vi "Get_Ini_File_Paths.vi"(2 "Error in":errorcluster) -> (0 "Error out":errorcluster)   [LabVIEW 2013]
uses:
  Globals/Ini_Files.vi
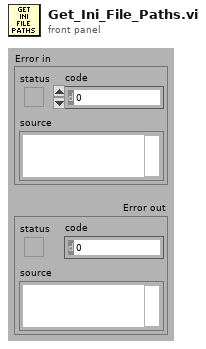
[diagram p1: front panel]
types:
  T1 = cluster{"Path Run Status file":path, "Path Default Settings file":path, "Path User Settings file":path}
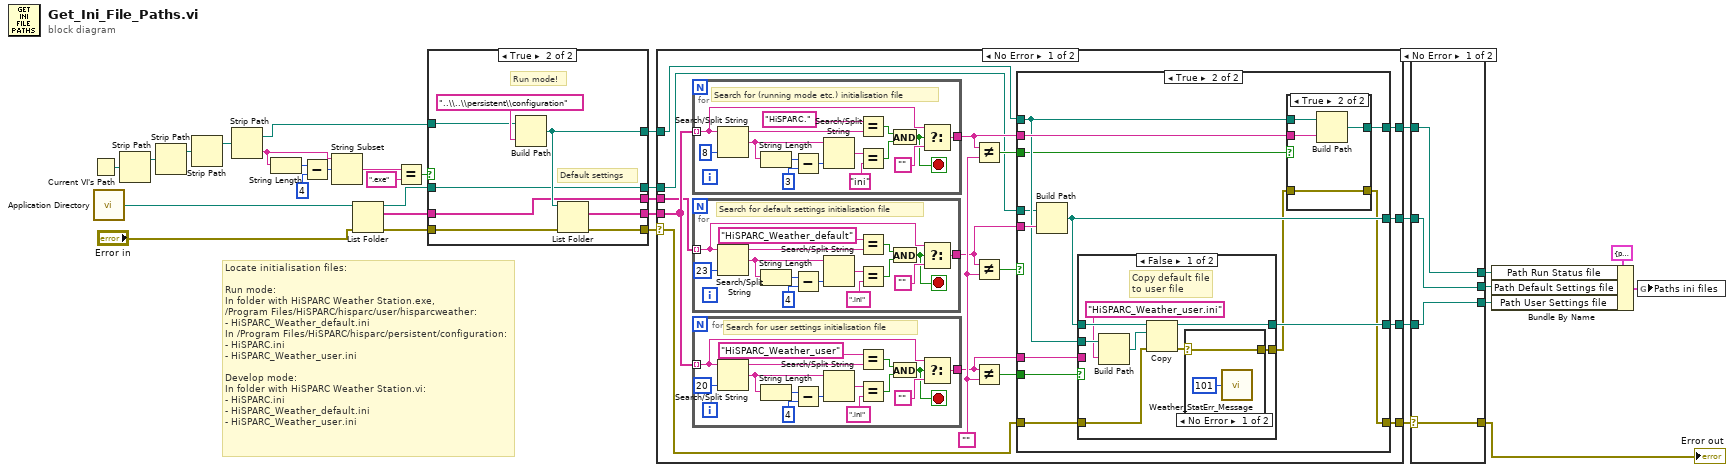
[diagram p0: block diagram]
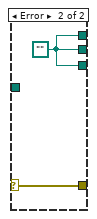
[diagram p3: hidden frame]
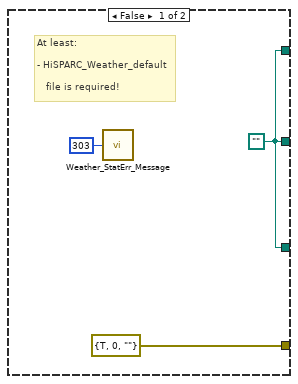
[diagram p4: hidden frame]
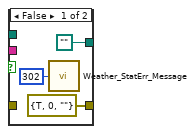
[diagram p5: hidden frame]
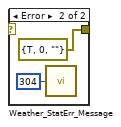
[diagram p6: hidden frame]
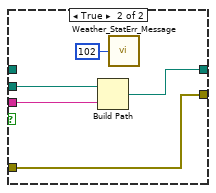
[diagram p7: hidden frame]
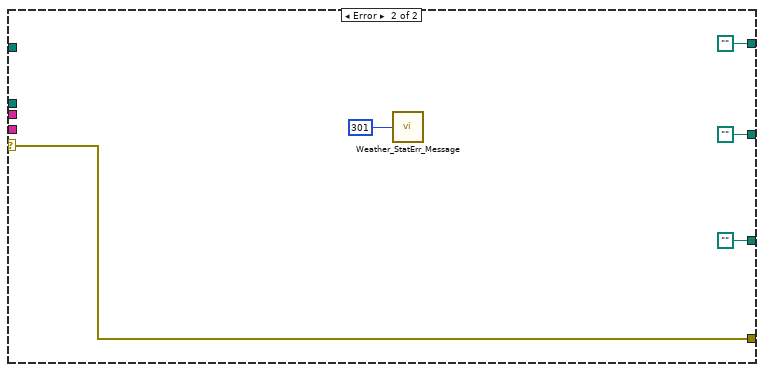
[diagram p8: hidden frame]
diagram:
  # "Locate initialisation files:\n\nRun mode:\nIn folder with HiSPARC Weather Station.exe,\n/Program Files/HiSPARC/hisparc/user/hisparcweather:\n- HiSPARC_Weather_default.ini\nIn /Program Files/HiSPARC/hisparc/persistent/configuration:\n- HiSPARC.ini\n- HiSPARC_Weather_user.ini\n\nDevelop mode:\nIn folder with HiSPARC Weather Station.vi:\n- HiSPARC.ini\n- HiSPARC_Weather_default.ini\n- HiSPARC_Weather_user.ini"
  n1 = Current VI's Path() -> (path=w7:path)
  n2 = call <vilib>:"Application Directory.vi"() -> ("Application Directory"=w8:path)
  n3 = Strip Path(path=w7) -> (stripped path=w6:path)  [unwired: 1 out]
  n4 = Strip Path(path=w6) -> (stripped path=w5:path)  [unwired: 1 out]
  n5 = Strip Path(path=w5) -> (stripped path=w3:path)  [unwired: 1 out]
  n6 = Strip Path(path=w3) -> (stripped path=w2:path, name=w4:string)
  n7 = String Length(string=w4) -> (length=w23:i32)
  n8 = Subtract(x=w23, y=4) -> (x-y=w21:i32)
  n9 = String Subset(string=w4, offset (0)=w21) -> (substring=w20:string)  [unwired: 1 in]
  n10 = List Folder(path=w8, error in="Error in") -> (path out=w15:path, filenames=w17:string[], error out=w14:errorcluster)  [unwired: 2 in, 1 out]
  n11 = Equal?(x=w20, y=".exe") -> (x = y?=w18:bool)
  n12 = case shown="True" w18 {
    tunnel: w17 -> [w33 w37]
    tunnel: w2 -> [_ w42]
    tunnel: w15 -> [w34 w39]
    tunnel: [w33 w36] -> w12
    tunnel: [w34 w39] -> w9
    tunnel: w14 -> [w35 w41]
    tunnel: [w35 w38] -> w13
    tunnel: [w34 w40] -> w10
    tunnel: [w33 w37] -> w11
    frame False {
      # "Develop mode!"
    }
    frame True {
      # "Default settings"
      # "Run mode!"
      n13 = Build Path(base path=w42, name or relative path="..\\..\\persistent\\configuration") -> (appended path=w40:path)
      n14 = List Folder(path=w40, error in=w41) -> (filenames=w36:string[], error out=w38:errorcluster)  [unwired: 2 in, 2 out]
    }
  }
  n15 = case shown="No Error" w13 {
    selector: w13 -> [w48 w146]
    tunnel: [w54 path "" ("Not A Path Constant")] -> w30
    tunnel: [w53 path ""] -> w32
    tunnel: [w52 path ""] -> w31
    tunnel: w12 -> [w47 _]
    tunnel: [w49 w146] -> w25
    tunnel: w11 -> [w46 _]
    tunnel: w10 -> [w45 _]
    tunnel: w9 -> [w44 _]
    frame No Error {
      w59 = ""
      n16 = for {
        tunnel: w47 -> [w92] mode=indexing
        tunnel: [w104] -> w56
        stop <- w93 stop-if-true
        # "Search for (running mode etc.) initialisation file"
        n17 = Search/Split String(string=w92, offset (0)=8 ("length (rest)")) -> (substring before match=w91:string, match + rest of string=w95:string)  [unwired: 2 out]
        n18 = String Length(string=w95) -> (length=w100:i32)
        n19 = Subtract(x=w100, y=3) -> (x-y=w98:i32)
        n20 = Search/Split String(string=w95, offset (0)=w98) -> (match + rest of string=w102:string)  [unwired: 1 in, 2 out]
        n21 = Equal?(x="HiSPARC." ("y"), y=w91) -> (x = y?=w94:bool)
        n22 = Equal?(x=w102, y="ini") -> (x = y?=w96:bool)
        n23 = And(x=w94, y=w96) -> (x .and. y?=w93:bool)
        n24 = Select(t=w92, s=w93, f="") -> (s? t:f=w104:string)
      }
      n25 = for {
        tunnel: w46 -> [w75] mode=indexing
        tunnel: [w89] -> w55
        stop <- w76 stop-if-true
        # "Search for default settings initialisation file"
        n26 = Search/Split String(string=w75, offset (0)=23 ("length (rest)")) -> (substring before match=w79:string, match + rest of string=w78:string)  [unwired: 2 out]
        n27 = String Length(string=w78) -> (length=w85:i32)
        n28 = Subtract(x=w85, y=4) -> (x-y=w83:i32)
        n29 = Search/Split String(string=w78, offset (0)=w83) -> (match + rest of string=w87:string)  [unwired: 1 in, 2 out]
        n30 = Equal?(x="HiSPARC_Weather_default" ("y"), y=w79) -> (x = y?=w77:bool)
        n31 = Equal?(x=w87, y=".ini") -> (x = y?=w81:bool)
        n32 = And(x=w77, y=w81) -> (x .and. y?=w76:bool)
        n33 = Select(t=w75, s=w76, f="") -> (s? t:f=w89:string)
      }
      n34 = for {
        tunnel: w47 -> [w74] mode=indexing
        tunnel: [w73] -> w57
        stop <- w60 stop-if-true
        # "Search for user settings initialisation file"
        n35 = Search/Split String(string=w74, offset (0)=20 ("length (rest)")) -> (substring before match=w63:string, match + rest of string=w62:string)  [unwired: 2 out]
        n36 = String Length(string=w62) -> (length=w69:i32)
        n37 = Subtract(x=w69, y=4) -> (x-y=w67:i32)
        n38 = Search/Split String(string=w62, offset (0)=w67) -> (match + rest of string=w71:string)  [unwired: 1 in, 2 out]
        n39 = Equal?(x="HiSPARC_Weather_user" ("y"), y=w63) -> (x = y?=w61:bool)
        n40 = Equal?(x=w71, y=".ini") -> (x = y?=w65:bool)
        n41 = And(x=w61, y=w65) -> (x .and. y?=w60:bool)
        n42 = Select(t=w74, s=w60, f="") -> (s? t:f=w73:string)
      }
      n43 = Not Equal?(x=w56, y=w59) -> (x != y?=w50:bool)
      n44 = Not Equal?(x=w55, y=w59) -> (x != y?=w51:bool)
      n45 = Not Equal?(x=w57, y=w59) -> (x != y?=w58:bool)
      n46 = case shown="True" w51 {
        tunnel: w58 -> [_ w120]
        tunnel: w57 -> [_ w118]
        tunnel: w56 -> [_ w116]
        tunnel: w55 -> [_ w115]
        tunnel: [w107 w117] -> w54
        tunnel: [w107 w112] -> w53
        tunnel: [w107 w119] -> w52
        tunnel: w45 -> [_ w114]
        tunnel: w50 -> [_ w113]
        tunnel: w48 -> [_ w111]
        tunnel: [errorcluster {"status"=TRUE, "code"=0, "source"=""} ("error IO") w110] -> w49
        tunnel: w44 -> [_ w108]
        frame False {
          w107 = path ""
          # "At least:\n\n- HiSPARC_Weather_default\n\n   file is required!"
          n47 = call "Weather_StatErr_Message.vi"("Message number"=303) -> ()  [unwired: 1 out]
        }
        frame True {
          n48 = Build Path(base path=w108, name or relative path=w115) -> (appended path=w112:path)
          n49 = case shown="False" w120 {
            tunnel: w114 -> [w133 w144]
            tunnel: [w135 w142] -> w119
            tunnel: w118 -> [_ w143]
            tunnel: w112 -> [w132 _]
            tunnel: w111 -> [w131 w141]
            tunnel: [w128 w141] -> w109
            frame False {
              # "Copy default file\nto user file"
              n50 = Build Path(base path=w133, name or relative path="HiSPARC_Weather_user.ini" ("y")) -> (appended path=w134:path)
              n51 = Copy(8:w131, 10:w134, 11:w132) -> (0:w129:errorcluster, 3:w135:path)  [unwired: 2 in, 1 out]
              n52 = case shown="No Error" w129 {
                selector: w129 -> [w137 _]
                tunnel: [w137 errorcluster {"status"=TRUE, "code"=0, "source"=""} ("error IO")] -> w128
                frame No Error {
                  n53 = call "Weather_StatErr_Message.vi"("Message number"=101) -> ()  [unwired: 1 out]
                }
                frame Error {
                  n54 = call "Weather_StatErr_Message.vi"("Message number"=304) -> ()  [unwired: 1 out]
                }
              }
            }
            frame True {
              n55 = Build Path(base path=w144, name or relative path=w143) -> (appended path=w142:path)
              n56 = call "Weather_StatErr_Message.vi"("Message number"=102) -> ()  [unwired: 1 out]
            }
          }
          n57 = case shown="True" w113 {
            tunnel: [path "" ("Not A Path Constant") w127] -> w117
            tunnel: w116 -> [_ w126]
            tunnel: w114 -> [_ w125]
            tunnel: [errorcluster {"status"=TRUE, "code"=0, "source"=""} ("error IO") w124] -> w110
            tunnel: w109 -> [_ w124]
            frame False {
              n58 = call "Weather_StatErr_Message.vi"("Message number"=302) -> ()  [unwired: 1 out]
            }
            frame True {
              n59 = Build Path(base path=w125, name or relative path=w126) -> (appended path=w127:path)
            }
          }
        }
      }
    }
    frame Error {
      n60 = call "Weather_StatErr_Message.vi"("Message number"=301) -> ()  [unwired: 1 out]
    }
  }
  n61 = case shown="No Error" w25 {
    selector: w25 -> [w150 w154]
    tunnel: w30 -> [w153 _]
    tunnel: w32 -> [w152 _]
    tunnel: w31 -> [w151 _]
    tunnel: [w153 w155] -> w28
    tunnel: [w152 w155] -> w27
    tunnel: [w151 w155] -> w26
    tunnel: [w150 w154] -> w24
    frame No Error {
    }
    frame Error {
      w155 = path ""
    }
  }
  "Error out" <- w24
  n62 = Bundle By Name(cluster=T1 {"Path Run Status file"=path "", "Path Default Settings file"=path "", "Path User Settings file"=path ""} ("input cluster"), "Path Run Status file"=w28, "Path Default Settings file"=w27, "Path User Settings file"=w26) -> (w1:T1)
  n63 = global write "Ini_Files.vi" "Paths ini files"(w1) -> ()
